vi "Drive Motors.vi"(11 "Cluster":T1) -> (2 "Left":cluster{"Left Motor Value":dbl, "output":dbl}(graph), 3 "Right":cluster{"Left Motor Value":dbl, "output":dbl}(graph))   [LabVIEW 2019]
uses:
  <vilib>/Rock Robotics/WPI/Utilities/WPI_GetSetVariantRefNum.vi
  Team Code/Robot Global Data.vi
  <vilib>/addons/control/pid/pid.llb/PID (DBL).vi
  <vilib>/Rock Robotics/Network Tables/SD Write Numeric Array.vi
  <vilib>/addons/control/pid/NI_PID_pid.lvlib
panel:
  in  "PID gains":T2={"proportional gain (Kc)"=1.0, "integral time (Ti, min)"=0.0, "derivative time (Td, min)"=0.0} {"derivative time (Td, min)" format="%.3f"; "integral time (Ti, min)" format="%.3f"; "proportional gain (Kc)" format="%.3f"}
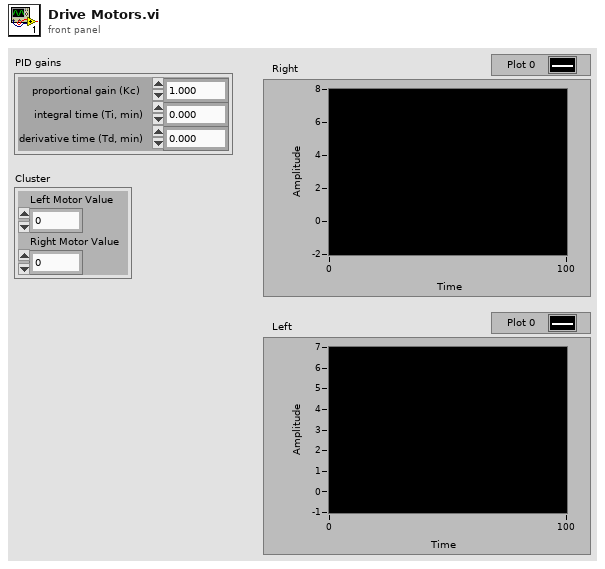
[diagram p1: front panel]
types:
  T1 = cluster{"Left Motor Value":dbl, "Right Motor Value":dbl}
  T2 = cluster{"proportional gain (Kc)":dbl, "integral time (Ti, min)":dbl, "derivative time (Td, min)":dbl}
  T3 = typedef "WPI_RobotDriveDevRef.ctl" = cluster{"DevStatus":errorcluster, "Motors[]":T4[], "Square Inputs":bool, "Max Output":dbl}
  T4 = typedef "WPI_MotorControlDeviceRef.ctl" = cluster{"DeviceStatus":errorcluster, "Type":T5, "PWM":cluster{"PWM Channel":T6, "DeadBand":T7}, "CAN":cluster{"Device Number":u8, "SetOutput VI Ref":variant, "GetOutput VI Ref":variant, "Enable VI Ref":variant, "Disable VI Ref":variant, "Data":variant}, "Invert":bool, "DIO PWM":cluster{"PWM \"Enable\" Channel":T6, "DIOChannel":T8, "PWM Rate":dbl}}
  T5 = typedef "WPI_MotorControlType.ctl" = enum16{"PWM", "CAN", "DIO PWM"}
  T6 = typedef "FPGA_DIOPWMChannel.ctl" = enum8{"PWM 0", "PWM 1", "PWM 2", "PWM 3", "PWM 4", "PWM 5", "PWM 6", "PWM 7", "PWM 8", "PWM 9", "PWM MXP 0", "PWM MXP 1", "PWM MXP 2", "PWM MXP 3", "PWM MXP 4", "PWM MXP 5", "PWM MXP 6", "PWM MXP 7", "PWM MXP 8", "PWM MXP 9", "Invalid"}
  T7 = typedef "WPI_PWMDeadband.ctl" = cluster{"Name":string, "maxPositivePwm":i32, "minPositivePwm":i32, "centerPwm":i32, "maxNegativePwm":i32, "minNegativePwm":i32, "angularRange":u16}
  T8 = typedef "FPGA_DIOChannel.ctl" = enum8{"DIO 0", "DIO 1", "DIO 2", "DIO 3", "DIO 4", "DIO 5", "DIO 6", "DIO 7", "DIO 8", "DIO 9", "DIO MXP 0", "DIO MXP 1", "DIO MXP 2", "DIO MXP 3", "DIO MXP 4", "DIO MXP 5", "DIO MXP 6", "DIO MXP 7", "DIO MXP 8", "DIO MXP 9", "DIO MXP 10", "DIO MXP 11", "DIO MXP 12", "DIO MXP 13", "DIO MXP 14", "DIO MXP 15", "SPI Port CS1", "SPI Port CS2", "SPI Port CS3", "SPI Port MISO", "SPI Port MOSI", "Invalid"}
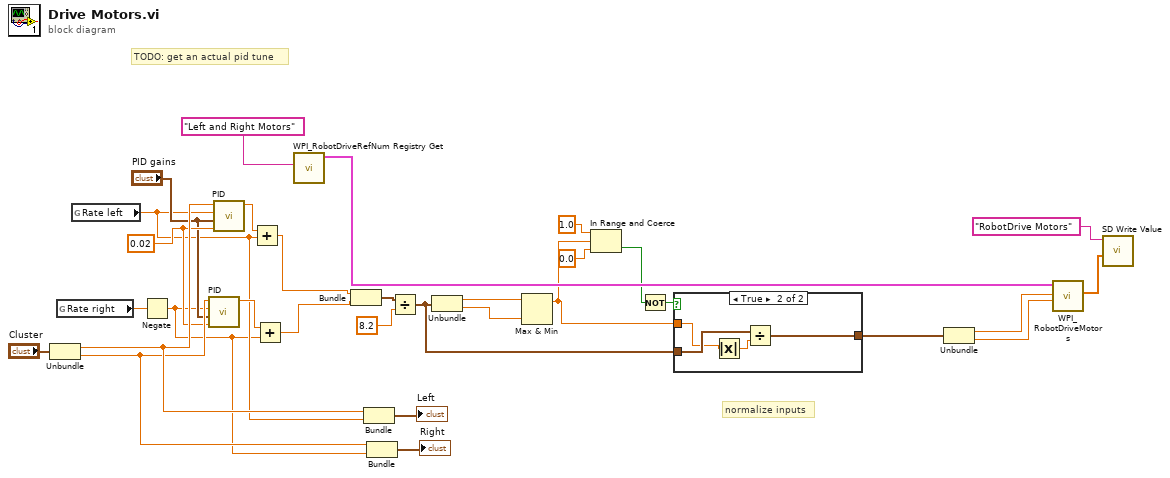
[diagram p0: block diagram]
diagram:
  w14 = 0.02 ("dt (s)")
  # "TODO: get an actual pid tune"
  # "normalize inputs"
  n1 = Unbundle("Cluster") -> ("Left Motor Value"=w30:dbl, "Right Motor Value"=w29:dbl)
  n2 = global read "Robot Global Data.vi" "Rate right"() -> (w2:dbl)
  n3 = global read "Robot Global Data.vi" "Rate left"() -> (w4:dbl)
  n4 = Negate(x=w2) -> (-x=w1:dbl)
  n5 = call-poly <vilib>:"PID.vi"("dt (s)"=w14, "PID gains"="PID gains", "process variable"=w1, "setpoint"=w29) -> ("output"=w25:dbl)  [unwired: 6 in, 1 out]
  n6 = call-poly <vilib>:"PID.vi"("dt (s)"=w14, "PID gains"="PID gains", "process variable"=w4, "setpoint"=w30) -> ("output"=w27:dbl)  [unwired: 6 in, 1 out]
  n7 = Add(x=w27, y=w4) -> (x+y=w28:dbl)
  n8 = Add(x=w25, y=w1) -> (x+y=w26:dbl)
  n9 = call <vilib>:"WPI_RobotDriveRefNum Registry Get.vi"("refnum name"="Left and Right Motors") -> ("RobotDriveDevRef"=w13:T3)  [unwired: 1 in, 9 out]
  n10 = Bundle(w28, w26) -> (w18:cluster{dbl, dbl})  [unwired: 1 in]
  n11 = Bundle("Left Motor Value"=w30, "Rate left"=w4) -> (→"Left":cluster{"Left Motor Value":dbl, "Rate left":dbl})  [unwired: 1 in]
  n12 = Bundle("Right Motor Value"=w29, w1) -> (→"Right":cluster{"Right Motor Value":dbl, dbl})  [unwired: 1 in]
  n13 = Divide(x=w18, y=8.2) -> (x/y=w22:cluster{dbl, dbl})
  n14 = Unbundle(w22) -> (w20:dbl, w21:dbl)
  n15 = Max & Min(x=w20, y=w21) -> (max(x,y)=w8:dbl)  [unwired: 1 out]
  n16 = In Range and Coerce(upper limit=1.0 ("x"), x=w8, lower limit=0.0 ("x")) -> (In Range?=w6:bool)  [unwired: 1 out]
  n17 = Not(x=w6) -> (.not. x?=w5:bool)
  n18 = case shown="True" w5 {
    tunnel: w8 -> [_ w34]
    tunnel: w22 -> [w32 w36]
    tunnel: [w32 w35] -> w31
    frame False {
    }
    frame True {
      n19 = Absolute Value(x=w34) -> (abs(x)=w33:dbl)
      n20 = Divide(x=w36, y=w33) -> (x/y=w35:cluster{dbl, dbl})
    }
  }
  n21 = Unbundle(w31) -> (w23:dbl, w24:dbl)
  n22 = call <vilib>:"WPI_RobotDriveMotors.vi"("RightSpeed"=w24, "LeftSpeed"=w23, "RobotDriveDevRef"=w13) -> ("Motor Values"=w16:dbl[])  [unwired: 6 in, 2 out]
  n23 = call-poly <vilib>:"SD Write Value.vi"("Numeric Array"=w16, "Name"="RobotDrive Motors") -> ()  [unwired: 8 in, 2 out]
